vi "2nd.vi"() -> ()   [LabVIEW 2016]
panel:
  out "Numeric 2":dbl
  out "Numeric":dbl
  in  "stop":bool
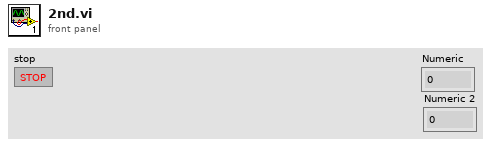
[diagram p1: front panel]
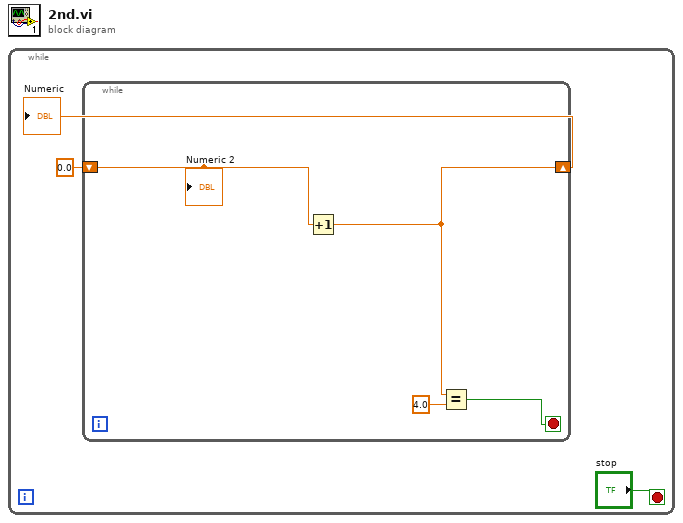
[diagram p0: block diagram]
diagram:
  n1 = while {
    stop <- "stop" stop-if-true
    n2 = while {
      shift-right: [w6] -> w1
      shift-left: 0.0 -> [w7]
      stop <- w4 stop-if-true
      n3 = Increment(x=w7) -> (x+1=w6:dbl)
      n4 = Equal?(x=w6, y=4.0) -> (x = y?=w4:bool)
      "Numeric 2" <- w7
    }
    "Numeric" <- w1
  }
